vi "Choreo_ReadTrajectoryFIle_Global_Example.vi"() -> ()   [LabVIEW 2019]
uses:
  SubVI/choreo_read_file_GlobalVariable.vi
  <vilib>/Rock Robotics/WPI/ThirdParty/ChoreoLib/ChoreoLib.lvlib
panel:
  out "error out":errorcluster
  # "Read Trajectory CSV File and \nWrite to Global Variable"
  # "See block diagram"
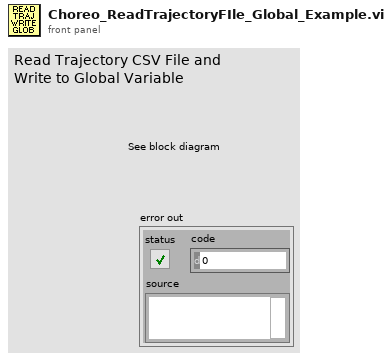
[diagram p1: front panel]
types:
  T1 = typedef "ChoreoLib.lvlib/ChoreoTrajectorySwerve.ctl" = cluster{"name":string, "samples":T2[], "splits":i32[], "events":T3[]}
  T2 = typedef "ChoreoLib.lvlib/ChoreoSwerveSample.ctl" = cluster{"timestamp":dbl, "x":dbl, "y":dbl, "heading":dbl, "velocityX":dbl, "velocityY":dbl, "angularVelocity":dbl, "accelX":dbl, "accelY":dbl, "accelAngular":dbl, "forceX":dbl[], "forceY":dbl[]}
  T3 = typedef "ChoreoLib.lvlib/ChoreoEventMarker.ctl" = cluster{"TimeStamp":dbl, "Name":string}
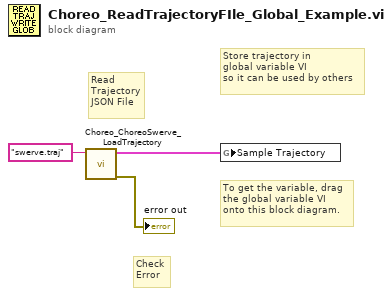
[diagram p0: block diagram]
diagram:
  # "Check\nError"
  # "Read\nTrajectory\nJSON File"
  # "To get the variable, drag\nthe global variable VI\nonto this block diagram."
  # "Store trajectory in\nglobal variable VI\nso it can be used by others"
  n1 = call <vilib>:"Choreo_ChoreoSwerve_LoadTrajectory.vi"("FileName"="swerve.traj" ("CSV File Name")) -> ("error out"=→"error out":errorcluster, "ChoreoTrajectorySwerve"=w2:T1)  [unwired: 8 in, 1 out]
  n2 = global write "choreo_read_file_GlobalVariable.vi" "Sample Trajectory"(w2) -> ()
